vi "SetDependenciesJKI.Robot.SMO.vi"(8 "error in (no error)":errorcluster, 10 "JKI.Robot":refnum<class "JKI.Robot.SMO.Base.lvclass">, 11 "JKI.Robot.SMO.APITesterUI in":refnum<class "JKI.Robot.SMO.APITesterUI.lvclass">) -> (0 "error out":errorcluster, 3 "JKI.Robot.SMO.APITesterUI out":refnum<class "JKI.Robot.SMO.APITesterUI.lvclass">)   [LabVIEW 2015, in "JKI.Robot.SMO.APITesterUI.lvclass"]
uses:
  JKI.Robot.SMO.APITesterUI.lvclass
  JKI.Robot.SMO.Base/JKI.Robot.SMO.Base.lvclass
  JKI.Robot.SMO.APITesterUI.lvclass/JKI.Robot.SMO.APITesterUI.ctl
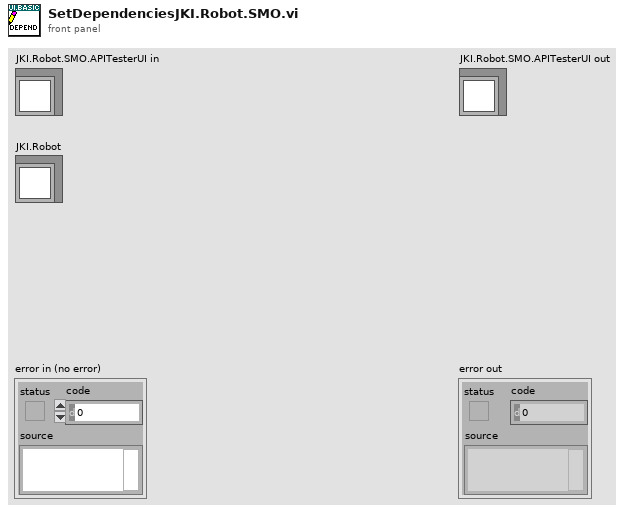
[diagram p1: front panel]
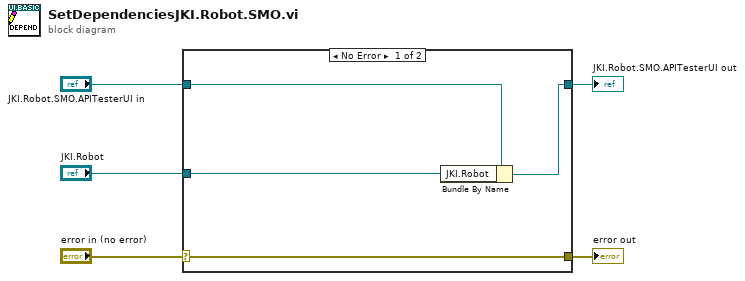
[diagram p0: block diagram]
diagram:
  n1 = case shown="No Error" "error in (no error)" {
    selector: "error in (no error)" -> [w9 w10]
    tunnel: [w9 w10] -> w4
    tunnel: [w7 w11] -> w2
    tunnel: "JKI.Robot.SMO.APITesterUI in" -> [w8 w11]
    tunnel: "JKI.Robot" -> [w6 _]
    frame No Error {
      n2 = Bundle By Name(cluster=w8, "JKI.Robot"=w6) -> (w7:refnum<class "JKI.Robot.SMO.APITesterUI.lvclass">)
    }
    frame Error {
    }
  }
  "error out" <- w4
  "JKI.Robot.SMO.APITesterUI out" <- w2
